vi "SimpleMotorFF_Pack__Ka_Tune_Params.vi"(8 "Ramp Rate":dbl, 9 "Max Eval SP":dbl, 10 "Min Eval SP":dbl, 11 "Max SP":dbl) -> (3 "Packed Params":T1)   [LabVIEW 2019, in "Trajectory_Library.lvlib"]
doc: "Pack individual parameters into the data cluster used by the Simple Motor Feed Forward Ka Auto Tune function. This function will ramp the SP up and down while collecting data. Once the ramp is complete Ka will be calculated.\n\nInputs: \n -- Max Sp -- Double -- The maximum value for the setpoint when ramping.\n -- Min Eval SP -- Double -- The lowest setpoint value to use when evaluating Ka\n -- Max Eval SP -- Double -- The highest setpoint value to use when evaluating Ka\n -- Ramp Rate -- Double -- The rate at which to ramp the setpoint (Units/Sec)\n\nOutputs:\n -- PackedParams -- SimpleMotorFF_KA_Tune_Params -- The packed data cluster."
uses:
  Trajectory_Library.lvlib
  TypeDef/SIMPLE_MOTOR_FF_KA_TUNE_PARAMS.ctl
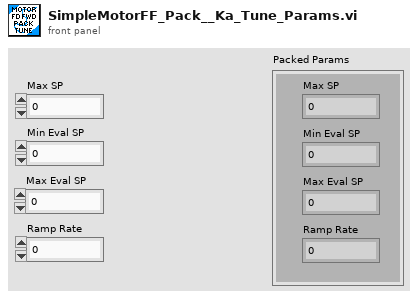
[diagram p1: front panel]
types:
  T1 = typedef "Trajectory_Library.lvlib/SIMPLE_MOTOR_FF_KA_TUNE_PARAMS.ctl" = cluster{"Max SP":dbl, "Min Eval SP":dbl, "Max Eval SP":dbl, "Ramp Rate":dbl}
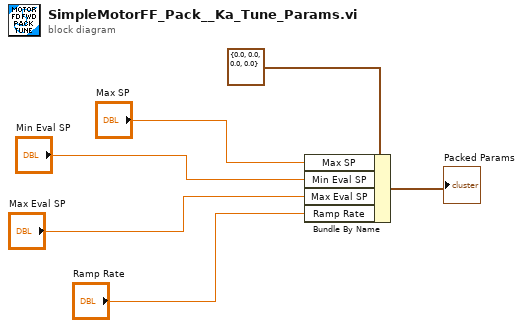
[diagram p0: block diagram]
diagram:
  n1 = Bundle By Name(cluster=T1 {"Max SP"=0.0, "Min Eval SP"=0.0, "Max Eval SP"=0.0, "Ramp Rate"=0.0} ("SimpleMotorFeedforward_KaTune_Pack"), "Max SP"="Max SP", "Min Eval SP"="Min Eval SP", "Max Eval SP"="Max Eval SP", "Ramp Rate"="Ramp Rate") -> (→"Packed Params":T1)
